vi "setCenterWavelength.vi"(6 "Delay between send and receive [ms]":i32=100, 8 "error in (no error)":errorcluster, 10 "wavelength":dbl, 11 "CCD in":refnum<class "CCD.lvclass">) -> (0 "error out":errorcluster, 1 "ID":i32, 2 "results-JSON string":string, 3 "CCD out":refnum<class "CCD.lvclass">)   [LabVIEW 2023, in "CCD.lvclass"]
doc: "This command sets the center wavelength value and other parameters to be used in the pixel to wavelength conversion.\n\nNote: This command should be called before ccd_setXAxisConversionType and ccd_setAcquisitionStart and is only useful uf the xAxisConversion type is set to Fitparams."
uses:
  CCD.lvclass
  CCD.lvclass/CCD.ctl
  20f7d3bd-08ac-4524-9bed-df36c1da25a0.vi
  GenericDevice/GenericDevice.lvclass
  a8db981f-de0e-4bb5-ae19-63df6e2f9c8d.vi
panel:
  # "Connector Pane"
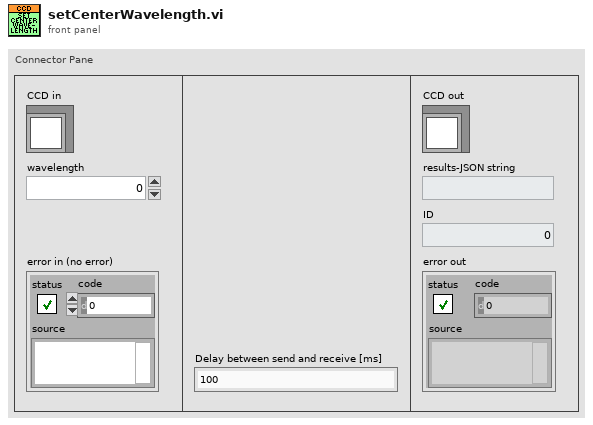
[diagram p1: front panel]
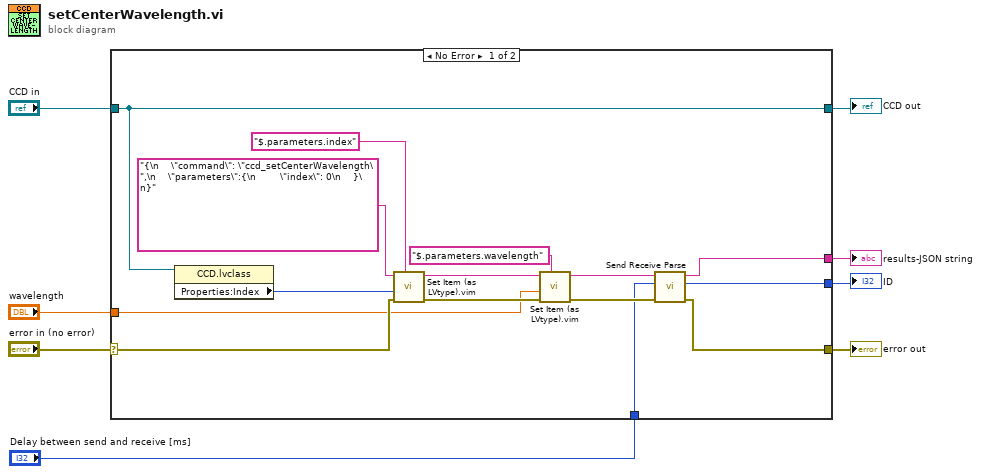
[diagram p0: block diagram]
diagram:
  n1 = case shown="No Error" "error in (no error)" {
    selector: "error in (no error)" -> [w19 w25]
    tunnel: [w12 w25] -> w7
    tunnel: [w21 w24] -> w5
    tunnel: "CCD in" -> [w21 w24]
    tunnel: "wavelength" -> [w9 _]
    tunnel: [w14 _] -> w4
    tunnel: [w13 _] -> w3
    tunnel: "Delay between send and receive [ms]" -> [w10 _]
    frame No Error {
      n2 = property class="CCD.lvclass"(reference=w21) -> ("Properties:Index"=w20:i32)  [unwired: 1 in, 2 out]
      n3 = call "Set Item (as LVtype).vim"("$Path or Item Name"="$.parameters.index", "error in (no error)"=w19, "Anything"=w20, "JSON"="{\n    \"command\": \"ccd_setCenterWavelength\",\n    \"parameters\":{\n        \"index\": 0\n    }\n}") -> ("error out"=w17:errorcluster, "<JSON>"=w18:string)  [unwired: 4 in, 1 out]
      n4 = call "Set Item (as LVtype).vim"("$Path or Item Name"="$.parameters.wavelength", "error in (no error)"=w17, "Anything"=w9, "JSON"=w18) -> ("error out"=w16:errorcluster, "<JSON>"=w11:string)  [unwired: 4 in, 1 out]
      n5 = call "Send Receive Parse.vi"("error in"=w16, "Delay between send and receive [ms]"=w10, "<JSON>"=w11) -> ("error out"=w12:errorcluster, "ID"=w13:i32, "results-JSON string"=w14:string)  [unwired: 6 in]
    }
    frame Error {
    }
  }
  "error out" <- w7
  "CCD out" <- w5
  "results-JSON string" <- w4
  "ID" <- w3
